vi "Init Getter.vi"(8 "error in (no error)":errorcluster, 9 "Getter Path":path, 10 "Class Type":refnum<class>, 11 "Binding in":refnum<class "Binding.lvclass">) -> (0 "error out":errorcluster, 3 "Binding out":refnum<class "Binding.lvclass">)   [LabVIEW 2020, in "PropertyBinder.lvlib" / "Binding.lvclass"]
uses:
  Binding.lvclass
  Getter Terminals.ctl
  Binding.lvclass/Binding.ctl
  PropertyBinder.lvlib
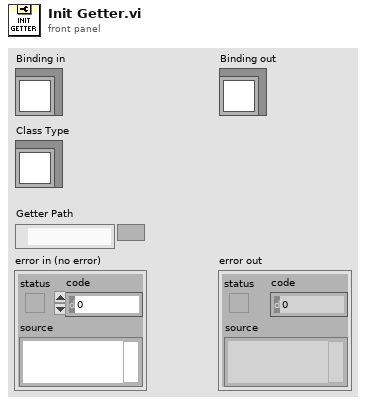
[diagram p1: front panel]
types:
  T1 = typedef "PropertyBinder.lvlib/Getter Terminals.ctl" = enum16{"Error out", "NC 1", "Value out", "Class out", "NC 4", "NC 5", "NC 6", "NC 7", "Error in", "NC 9", "NC 10", "Class in"}
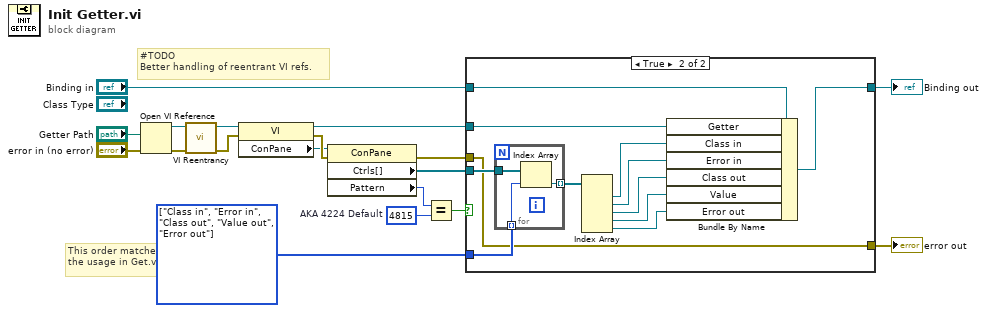
[diagram p0: block diagram]
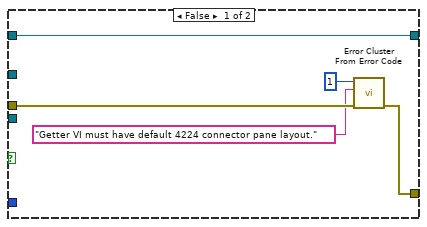
[diagram p2: hidden frame]
diagram:
  w8 = T1[] [enum."Class in", enum."Error in", enum."Class out", enum."Value out", enum."Error out"] items=["Error out", "NC 1", "Value out", "Class out", "NC 4", "NC 5", "NC 6", "NC 7", "Error in", "NC 9", "NC 10", "Class in"]
  w12 = u32 4815  # AKA 4224 Default
  # "This order matches the usage in Get.vi"
  # "#TODO\nBetter handling of reentrant VI refs."
  n1 = Open VI Reference(vi path="Getter Path", error in (no error)="error in (no error)") -> (vi reference=w16:refnum<vi>, error out=w15:errorcluster)  [unwired: 4 in]
  n2 = call "VI Reentrancy.vi"("error in (no error)"=w15, "VI in"=w16) -> ("error out"=w4:errorcluster, "VI"=w14:refnum<vi>)  [unwired: 7 in, 1 out]
  n3 = property class="VI"(reference=w14, error in=w4) -> (reference out=w7:refnum<vi>, error out=w18:errorcluster, "ConPane"=w11:refnum<vi>)
  n4 = property class="ConPane"(reference=w11, error in=w18) -> (error out=w3:errorcluster, "Ctrls[]"=w9:refnum<vi>[], "Pattern"=w13:u32)  [unwired: 1 out]
  n5 = Equal?(x=w13, y=w12) -> (x = y?=w10:bool)
  n6 = case shown="True" w10 {
    tunnel: w9 -> [_ w35]
    tunnel: w8 -> [_ w34]
    tunnel: w7 -> [_ w29]
    tunnel: "Binding in" -> [w23 w33]
    tunnel: [w23 w32] -> w5
    tunnel: w3 -> [w22 w30]
    tunnel: [w19 w30] -> w1
    frame False {
      n7 = call <vilib>:"Error Cluster From Error Code.vi"("error in (no error)"=w22, "error message (\"\")"="Getter VI must have default 4224 connector pane layout." ("error message (\"\")"), "error code (0)"=1) -> ("error out"=w19:errorcluster)  [unwired: 6 in]
    }
    frame True {
      n8 = for {
        tunnel: w35 -> [w38]
        tunnel: w34 -> [w37] mode=indexing
        tunnel: [w36] -> w31 mode=indexing
        n9 = Index Array(array=w38, index=w37) -> (element=w36:refnum<vi>)
      }
      n10 = Index Array(array=w31) -> (element #1=w28:refnum<vi>, element #2=w27:refnum<vi>, element #3=w26:refnum<vi>, element #4=w25:refnum<vi>, element #5=w24:refnum<vi>)  [unwired: 5 in]
      n11 = Bundle By Name(cluster=w33, "Getter"=w29, "Class in"=w28, "Error in"=w27, "Class out"=w26, "Value"=w25, "Error out"=w24) -> (w32:refnum<class "Binding.lvclass">)
    }
  }
  "error out" <- w1
  "Binding out" <- w5
